vi "input-validation_v3.vi"(8 "error constant":errorcluster, 9 "Ki-xy":sgl=0.005, 11 "z_axis_params":T1={"TOL"=0.3, "ramp_rate"=-5e-06, "z_u_max"=5.0, "setpoint"=0.0, "Ki"=0.001, "Z_error_threshold"=0.0, "Z_settled_samples_threshold "=0, "zup_rate"=0.0, "uz_safe"=0.0, "Kiz_down"=0.001, "max_Z_settle_samples"=5000} {"uz_safe" format="%#_13g"; "Z_error_threshold" format="%#_13g"; "ramp_rate" format="%#_4g"; "TOL" format="%#_13g"}) -> (0 "error out":errorcluster)   [LabVIEW 2017]
uses:
  controls/z-axis-params_v3.ctl
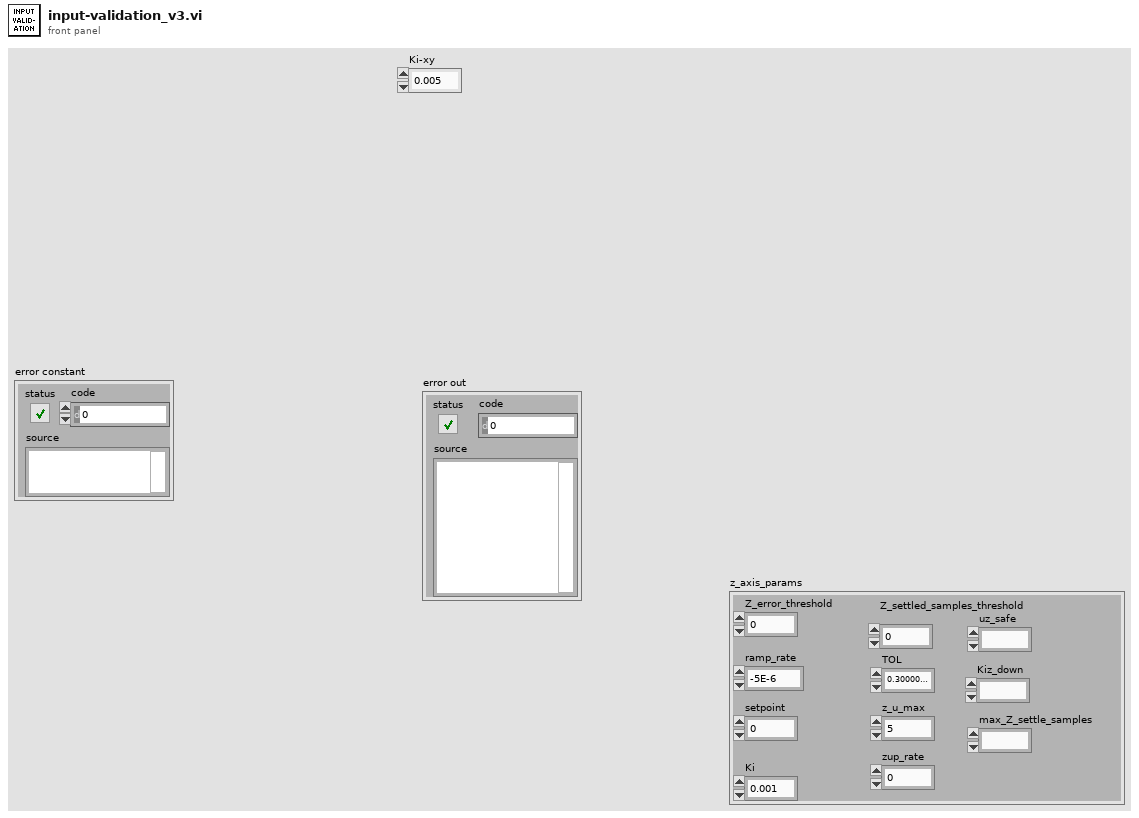
[diagram p1: front panel]
types:
  T1 = typedef "z-axis-params_v3.ctl" = cluster{"TOL":sgl, "ramp_rate":sgl, "z_u_max":sgl, "setpoint":sgl, "Ki":sgl, "Z_error_threshold":sgl, "Z_settled_samples_threshold ":i16, "zup_rate":sgl, "uz_safe":fxp<+/-,16,5>, "Kiz_down":sgl, "max_Z_settle_samples":i16}
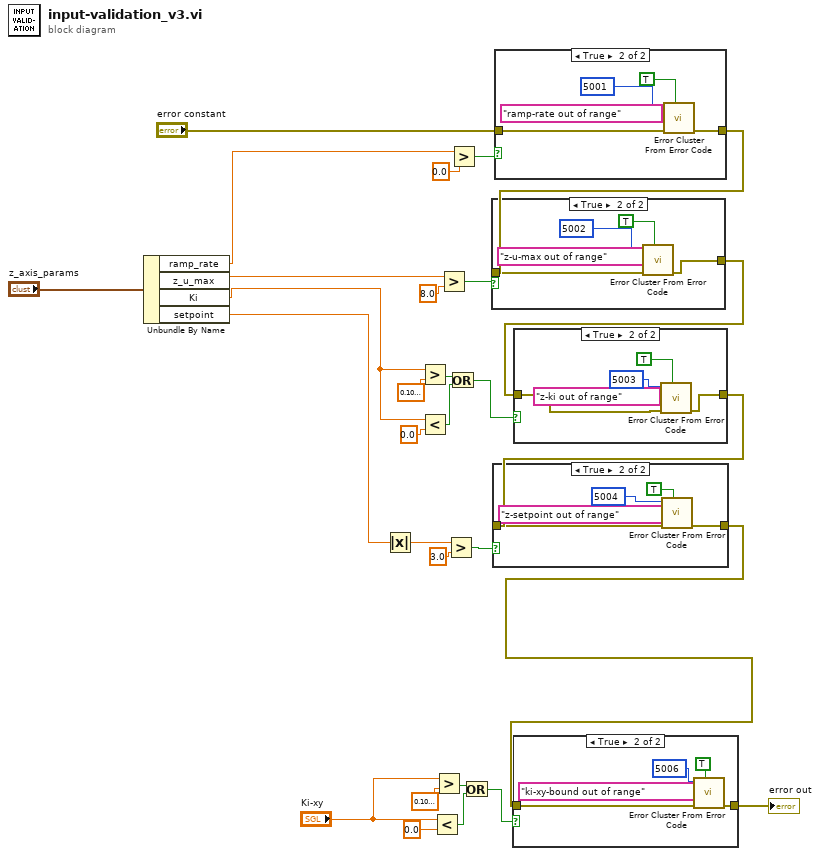
[diagram p0: block diagram]
diagram:
  n1 = Unbundle By Name("z_axis_params") -> ("ramp_rate"=w24:sgl, "z_u_max"=w22:sgl, "Ki"=w4:sgl, "setpoint"=w3:sgl)
  n2 = Absolute Value(x=w3) -> (abs(x)=w28:sgl)
  n3 = Greater?(x=w4, y=sgl 0.1) -> (0:w13:bool)
  n4 = Less?(x=w4, y=sgl 0.0) -> (x < y?=w14:bool)
  n5 = Less?(x="Ki-xy", y=sgl 0.0) -> (x < y?=w8:bool)
  n6 = Greater?(x="Ki-xy", y=sgl 0.1) -> (0:w9:bool)
  n7 = Greater?(x=w22, y=sgl 8.0) -> (0:w11:bool)
  n8 = Greater?(x=w28, y=sgl 3.0) -> (0:w15:bool)
  n9 = Or(x=w13, y=w14) -> (x .or. y?=w12:bool)
  n10 = Greater?(x=w24, y=sgl 0.0) -> (0:w19:bool)
  n11 = Or(x=w9, y=w8) -> (x .or. y?=w7:bool)
  n12 = case shown="True" w19 {
    tunnel: "error constant" -> [w30 w35]
    tunnel: [w30 w31] -> w18
    frame False {
    }
    frame True {
      n13 = call <vilib>:"Error Cluster From Error Code.vi"("show call chain? (False)"=TRUE, "error in (no error)"=w35, "error message (\"\")"="ramp-rate out of range", "error code (0)"=5001) -> ("error out"=w31:errorcluster)  [unwired: 5 in]
    }
  }
  n14 = case shown="True" w11 {
    tunnel: w18 -> [w36 w39]
    tunnel: [w36 w40] -> w17
    frame False {
    }
    frame True {
      n15 = call <vilib>:"Error Cluster From Error Code.vi"("show call chain? (False)"=TRUE, "error in (no error)"=w39, "error message (\"\")"="z-u-max out of range", "error code (0)"=5002) -> ("error out"=w40:errorcluster)  [unwired: 5 in]
    }
  }
  n16 = case shown="True" w12 {
    tunnel: w17 -> [w42 w43]
    tunnel: [w42 w44] -> w16
    frame False {
    }
    frame True {
      n17 = call <vilib>:"Error Cluster From Error Code.vi"("show call chain? (False)"=TRUE, "error in (no error)"=w43, "error message (\"\")"="z-ki out of range", "error code (0)"=5003) -> ("error out"=w44:errorcluster)  [unwired: 5 in]
    }
  }
  n18 = case shown="True" w15 {
    tunnel: w16 -> [w48 w51]
    tunnel: [w48 w52] -> w1
    frame False {
    }
    frame True {
      n19 = call <vilib>:"Error Cluster From Error Code.vi"("show call chain? (False)"=TRUE, "error in (no error)"=w51, "error message (\"\")"="z-setpoint out of range", "error code (0)"=5004) -> ("error out"=w52:errorcluster)  [unwired: 5 in]
    }
  }
  n20 = case shown="True" w7 {
    tunnel: [w54 w56] -> w2
    tunnel: w1 -> [w54 w57]
    frame False {
    }
    frame True {
      n21 = call <vilib>:"Error Cluster From Error Code.vi"("show call chain? (False)"=TRUE, "error in (no error)"=w57, "error message (\"\")"="ki-xy-bound out of range", "error code (0)"=5006) -> ("error out"=w56:errorcluster)  [unwired: 5 in]
    }
  }
  "error out" <- w2
